vi "turn.vi"(5 "Angle":dbl, 7 "side":enum16{"right", "left"}(ring), 8 "error in (no error)":errorcluster, 11 "KNR in":T1) -> (0 "error out":errorcluster, 3 "KNR out":T1)   [LabVIEW 2013]
uses:
  <userlib>/KNR OS 3.0 LabVIEW Toolkit/Type Definition/KNR3 Reference.ctl
  <userlib>/_FPGA Interface Advanced Tools/FPGA Interface Base/FPGA Interface Base.lvclass
  <userlib>/KNR OS 3.0 LabVIEW Toolkit/Type Definition/Resource.ctl
  Global 1.vi
panel:
  out "move 2":i32
  out "after right 2":i32
  out "after left 2":i32
  out "move":i32
  out "after left":i32
  out "position right":i32
  out "after right":i32
  out "should move":i32
  out "position left":i32
  in  "left":bool
  in  "right":bool
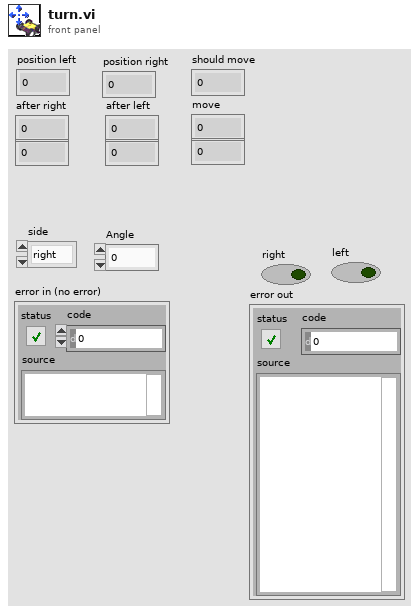
[diagram p1: front panel]
types:
  T1 = typedef "KNR3 Reference.ctl" = cluster{"FPGA Session":refnum<class "FPGA Interface Base.lvclass">, "Resource":T2}
  T2 = typedef "Resource.ctl" = enum16{"KNRm_DDRC", "KNRm_DDDD", "KNRm_DDDR", "KNRm_DDDC", "KNR"}
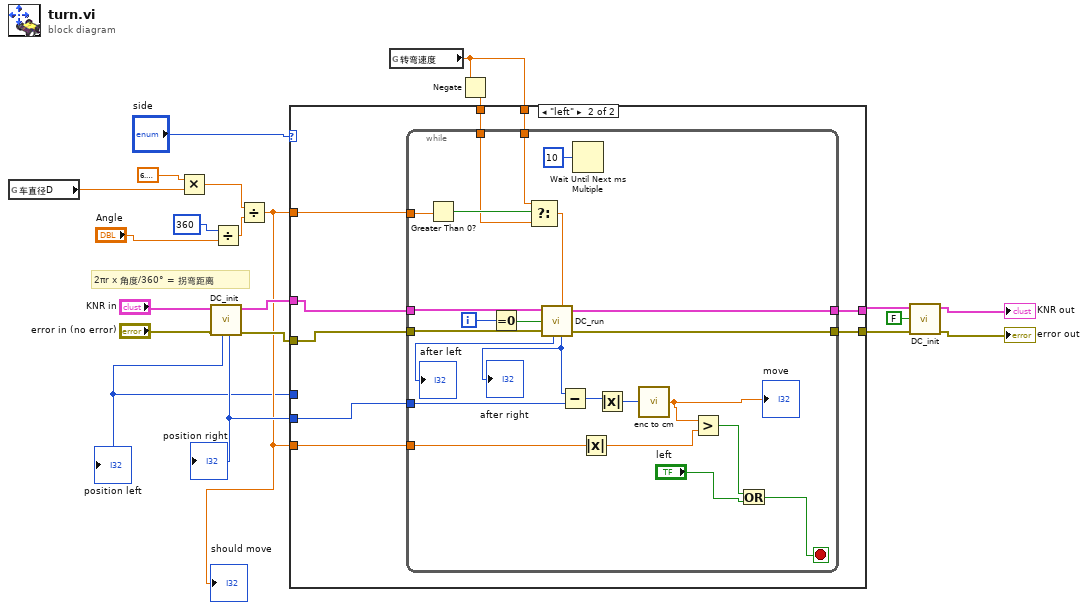
[diagram p0: block diagram]
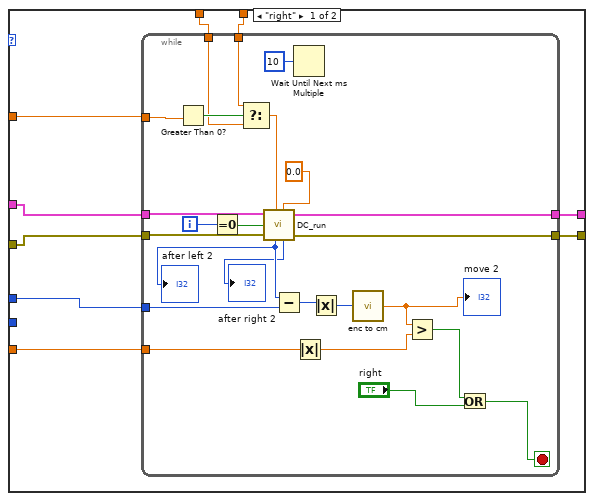
[diagram p2: hidden frame]
diagram:
  # "2πr x 角度/360° = 拐弯距离"
  n1 = global read "Global 1.vi" "车直径D"() -> (w3:dbl)
  n2 = Multiply(x=6.283185307179586, y=w3) -> (x*y=w19:dbl)
  n3 = call "DC_init.vi"("error in (no error)"="error in (no error)", "KNR in"="KNR in") -> ("error out"=w9:errorcluster, "KNR out"=w10:T1, "output\nposition 2"=w6:i32, "output\nPosition_1"=w4:i32)  [unwired: 6 in]
  "position left" <- w4
  "position right" <- w6
  n4 = Divide(x=360, y="Angle") -> (x/y=w18:dbl)
  n5 = Divide(x=w19, y=w18) -> (x/y=w5:dbl)
  "should move" <- w5
  n6 = global read "Global 1.vi" "转弯速度"() -> (w1:dbl)
  n7 = Negate(x=w1) -> (-x=w2:dbl)
  n8 = case shown="\"left\"" "side" {
    tunnel: w5 -> [w30 w61]
    tunnel: [w29 w60] -> w15
    tunnel: [w28 w59] -> w14
    tunnel: w10 -> [w27 w62]
    tunnel: w9 -> [w26 w63]
    tunnel: w6 -> [_ w58]
    tunnel: w5 -> [w24 w57]
    tunnel: w4 -> [w25 _]
    tunnel: w1 -> [w23 w56]
    tunnel: w2 -> [w22 w55]
    frame "right" {
      n9 = while {
        tunnel: w30 -> [w39]
        tunnel: w27 -> [w52]
        tunnel: w26 -> [w51]
        tunnel: [w43] -> w29
        tunnel: [w42] -> w28
        tunnel: w25 -> [w40]
        tunnel: w24 -> [w36]
        tunnel: w23 -> [w32]
        tunnel: w22 -> [w31]
        i -> [w50]
        stop <- w41 stop-if-true
        n10 = Greater Than 0?(x=w39) -> (x > 0?=w54:bool)
        n11 = Equal To 0?(x=w50) -> (x = 0?=w49:bool)
        n12 = Select(t=w32, s=w54, f=w31) -> (s? t:f=w44:dbl)
        n13 = call "DC_run.vi"("KNR in"=w52, "speed_1"=w44, "reinitialize? (F)"=w49, "error in (no error)"=w51, "speed_2"=0.0) -> ("Position_1"=w35:i32, "KNR out"=w43:T1, "Position_2"=→"after right 2":i32, "error out"=w42:errorcluster)  [unwired: 1 in]
        "after left 2" <- w35
        n14 = Subtract(x=w35, y=w40) -> (x-y=w48:i32)
        n15 = Wait Until Next ms Multiple(millisecond multiple=u32 10) -> ()  [unwired: 1 out]
        n16 = Absolute Value(x=w36) -> (abs(x)=w47:dbl)
        n17 = Absolute Value(x=w48) -> (abs(x)=w45:i32)
        n18 = call "enc to cm.vi"("E"=w45) -> ("CM"=w33:dbl)  [unwired: 1 in]
        "move 2" <- w33
        n19 = Greater?(x=w33, y=w47) -> (0:w46:bool)
        n20 = Or(x=w46, y="right") -> (x .or. y?=w41:bool)
      }
    }
    frame "left" {
      n21 = while {
        tunnel: w61 -> [w71]
        tunnel: w62 -> [w84]
        tunnel: w63 -> [w83]
        tunnel: [w75] -> w60
        tunnel: [w74] -> w59
        tunnel: w58 -> [w72]
        tunnel: w57 -> [w69]
        tunnel: w56 -> [w65]
        tunnel: w55 -> [w64]
        i -> [w82]
        stop <- w76 stop-if-true
        n22 = Greater Than 0?(x=w71) -> (x > 0?=w86:bool)
        n23 = Equal To 0?(x=w82) -> (x = 0?=w81:bool)
        n24 = Select(t=w65, s=w86, f=w64) -> (s? t:f=w73:dbl)
        n25 = call "DC_run.vi"("KNR in"=w84, "reinitialize? (F)"=w81, "error in (no error)"=w83, "speed_2"=w73) -> ("Position_1"=→"after left":i32, "KNR out"=w75:T1, "Position_2"=w67:i32, "error out"=w74:errorcluster)  [unwired: 2 in]
        "after right" <- w67
        n26 = Subtract(x=w67, y=w72) -> (x-y=w80:i32)
        n27 = Wait Until Next ms Multiple(millisecond multiple=u32 10) -> ()  [unwired: 1 out]
        n28 = Absolute Value(x=w69) -> (abs(x)=w79:dbl)
        n29 = Absolute Value(x=w80) -> (abs(x)=w77:i32)
        n30 = call "enc to cm.vi"("E"=w77) -> ("CM"=w66:dbl)  [unwired: 1 in]
        "move" <- w66
        n31 = Greater?(x=w66, y=w79) -> (0:w78:bool)
        n32 = Or(x=w78, y="left") -> (x .or. y?=w76:bool)
      }
    }
  }
  n33 = call "DC_init.vi"("error in (no error)"=w14, "Enable Motor(T)"=FALSE, "KNR in"=w15) -> ("error out"=→"error out":errorcluster, "KNR out"=→"KNR out":T1)  [unwired: 5 in, 2 out]
